vi "Median Filter.vi"(9 "right rank":i32=-1, 10 "left rank":i32=2, 11 "X":dbl[](array[numeric])) -> (0 "error":i32, 3 "Filtered X":dbl[](array[numeric]))   [LabVIEW 2020, in "NI_AALBase.lvlib"]
doc: "Applies a median filter of rank to the input sequence <B>X</B>."
uses:
  <vilib>/Analysis/NI_AALBase.lvlib
  <resource>/lvanlys.dll
panel:
  # "Median Filter"
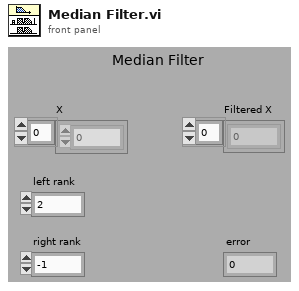
[diagram p1: front panel]
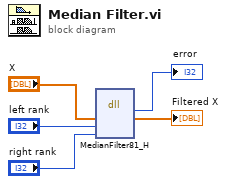
[diagram p0: block diagram]
diagram:
  n1 = dll-call lib="e:/builds/penguin/labview/branches/2020/dev/dist/resource/lvanlys.*" fn="MedianFilter81_H"("xHandle"="X", "left rank"="left rank", "right rank"="right rank") -> (→"error":i32, "xHandle"=→"Filtered X":dbl[])  [unwired: 5 in, 2 out]
